vi "Init_Devices.vi"(8 "error in":errorcluster) -> (0 "error out":errorcluster, 2 "Error string":string)   [LabVIEW 2021]
uses:
  Arduino serial init/ard_RS232_states.ctl
  RS485 serial init/RS485_RS232_states.ctl
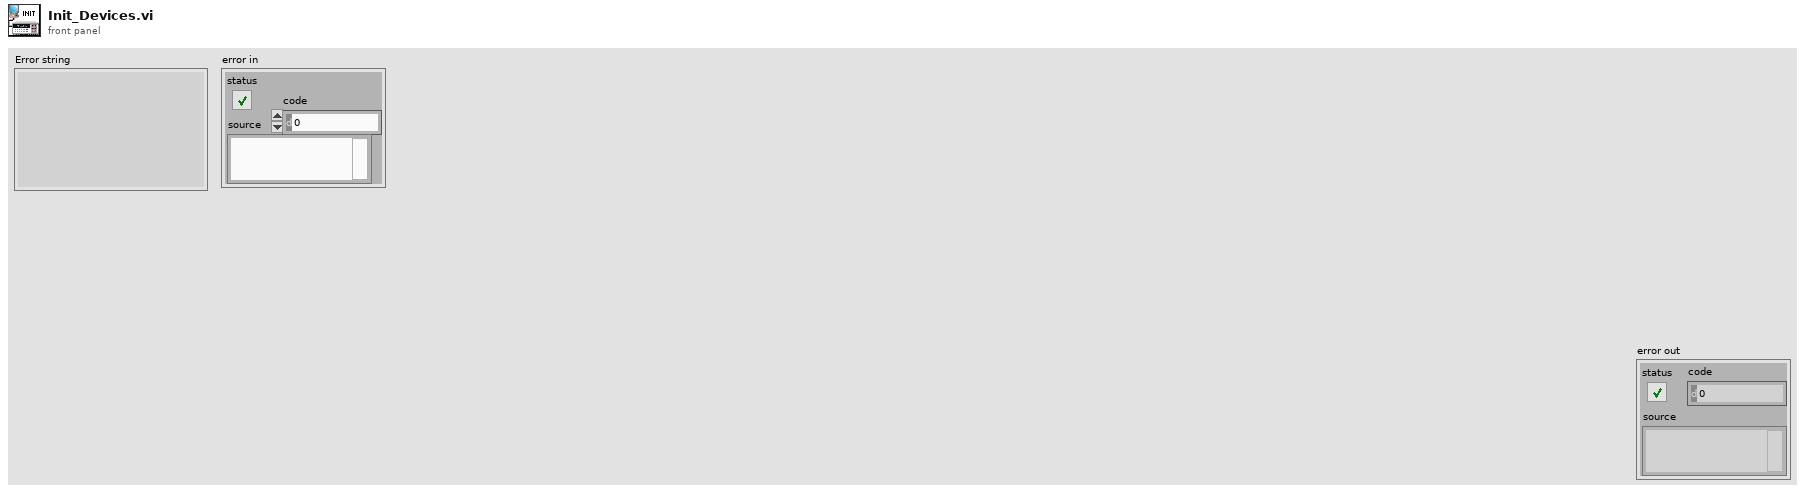
[diagram p1: front panel]
types:
  T1 = typedef "RS485_RS232_states.ctl" = enum16{"Init", "Read", "Write", "Clear", "Close", "Write&Read"}
  T2 = typedef "ard_RS232_states.ctl" = enum16{"Init", "Read", "Write", "Clear", "Close", "Write&Read"}
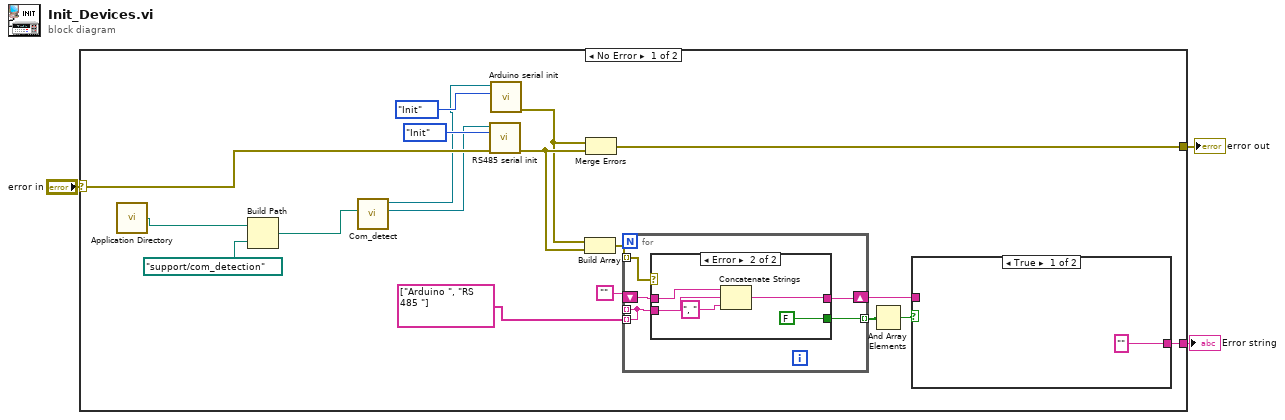
[diagram p0: block diagram]
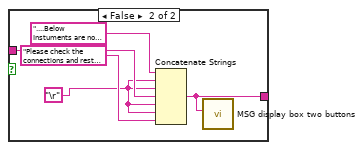
[diagram p2: hidden frame]
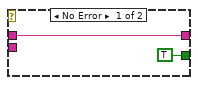
[diagram p3: hidden frame]
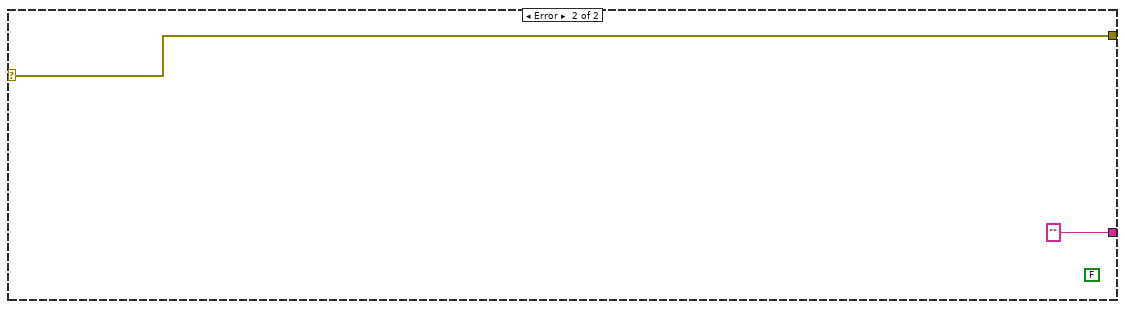
[diagram p4: hidden frame]
diagram:
  n1 = case shown="No Error" "error in" {
    selector: "error in" -> [w16 w41]
    tunnel: [w18 w41] -> w3
    tunnel: [w13 ""] -> w1
    frame No Error {
      n2 = call <vilib>:"Application Directory.vi"() -> ("Application Directory"=w5:path)
      n3 = Build Path(base path=w5, name or relative path=path "support/com_detection") -> (appended path=w9:path)
      n4 = call "Com_detect.vi"("Application Directory"=w9) -> ("RS485_1"=w11:refnum<visa-resource-name>, "Ardu"=w12:refnum<visa-resource-name>)  [unwired: 8 in, 1 out]
      n5 = call "RS485 serial init .vi"("error in"=w16, "RS232_State"=RS485_RS232_states."Init", "Resource Name"=w11) -> ("error out"=w17:errorcluster)  [unwired: 5 in, 3 out]
      n6 = call "Arduino serial init .vi"("RS232_State"=ard_RS232_states."Init", "Resource Name"=w12) -> ("error out"=w8:errorcluster)  [unwired: 6 in, 3 out]
      n7 = Build Array(w8, w17) -> (w21:errorcluster[])
      n8 = Merge Errors(w8, w17) -> (w18:errorcluster)
      n9 = for {
        tunnel: w21 -> [w30] mode=indexing
        tunnel: [w28] -> _ mode=indexing
        shift-right: [w31] -> w19
        shift-left: "" -> [w32]
        tunnel: [w29] -> w7 mode=indexing
        tunnel: string[] ["Arduino ", "RS 485 "] -> [w28] mode=indexing
        n10 = case shown="Error" w30 {
          tunnel: w28 -> [_ w38]
          tunnel: w32 -> [w34 w39]
          tunnel: [w34 w36] -> w31
          tunnel: [TRUE FALSE] -> w29
          frame No Error {
          }
          frame Error {
            n11 = Concatenate Strings(w39, w38, ", " ("string")) -> (w36:string)
          }
        }
      }
      n12 = And Array Elements(Boolean array=w7) -> (logical AND=w6:bool)
      n13 = case shown="True" w6 {
        tunnel: w19 -> [_ w27]
        tunnel: ["" w23] -> w13
        frame True {
        }
        frame False {
          w24 = "\r"
          n14 = Concatenate Strings("....Below Instuments are not properly initialised..." ("Initial Message"), w24, w24, w27, w24, w24, "Please check the connections and restart the application" ("Initial Message")) -> (w23:string)
          n15 = call "MSG display box two buttons.vi"("input string"=w23) -> ()  [unwired: 9 in, 2 out]
        }
      }
    }
    frame Error {
      (unwired) FALSE ("OK Button 2")
    }
  }
  "error out" <- w3
  "Error string" <- w1
